vi "HasCursorPosChanged.vi"(1 "Decay reference":refnum<vi>) -> (0 "changed?":bool)   [LabVIEW 2009]
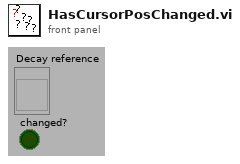
[diagram p1: front panel]
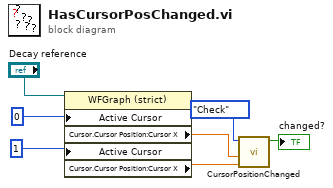
[diagram p0: block diagram]
diagram:
  n1 = property class="WFGraph (strict)"(reference="Decay reference", "Active Cursor"=u32 0, "Active Cursor"=u32 1) -> ("Cursor.Cursor Position:Cursor X"=w4:dbl, "Cursor.Cursor Position:Cursor X"=w3:dbl)  [unwired: 1 in, 2 out]
  n2 = call "CursorPositionChanged.vi"("CursorPos x1"=w3, "CursorPos x0"=w4, "action"=enum16{"Check", "Get", "xval"}."Check" ("Enum")) -> ("cursorpos changed?"=→"changed?":bool)  [unwired: 1 in, 3 out]
